vi "Interlock Chain Close Connections.vi"(8 "error in (no error)":errorcluster, 11 "CO2 Actor in":refnum<class "CO2 Actor.lvclass">) -> (0 "error out":errorcluster, 3 "CO2 Actor out":refnum<class "CO2 Actor.lvclass">)   [LabVIEW 2015, in "cRIO-Carbondioxide.lvlib" / "CO2-Actor.lvlib" / "CO2 Actor.lvclass"]
uses:
  CO2 Actor.lvclass
  CO2 Actor.lvclass/CO2 Actor.ctl
  Interlocks/Interlock Chain/Interlock Chain.lvclass/Interlock Chain.ctl
  Interlocks/Interlock/Interlock.lvclass
  Interlocks/Interlock Chain/Interlock Chain.lvclass
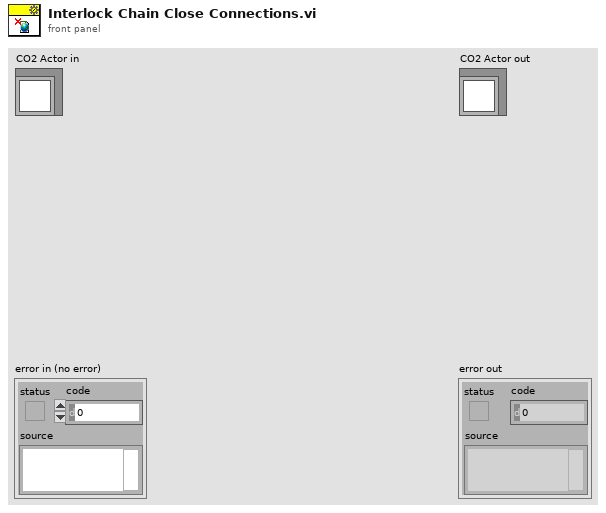
[diagram p1: front panel]
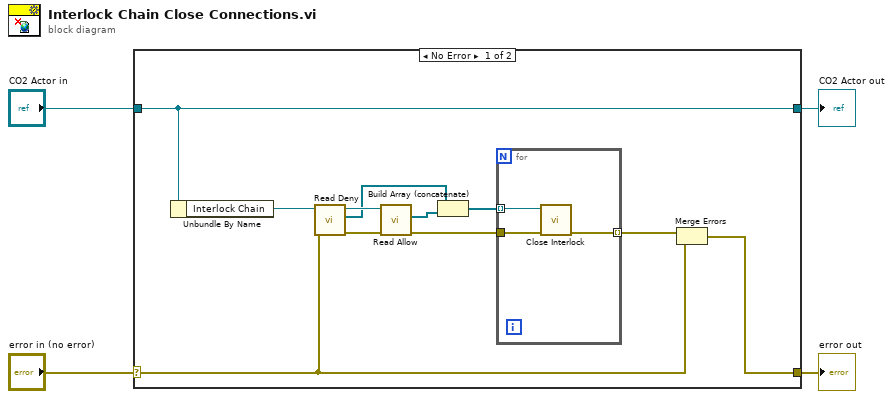
[diagram p0: block diagram]
diagram:
  n1 = case shown="No Error" "error in (no error)" {
    selector: "error in (no error)" -> [w11 w20]
    tunnel: [w13 w20] -> w3
    tunnel: [w15 w19] -> w1
    tunnel: "CO2 Actor in" -> [w15 w19]
    frame No Error {
      n2 = Unbundle By Name(w15) -> ("Interlock Chain"=w12:refnum<class "Interlock Chain.lvclass">)
      n3 = call "Read Deny.vi"("error in (no error)"=w11, "Interlock Chain in"=w12) -> ("error out"=w10:errorcluster, "Deny"=w5:refnum<class "Interlock.lvclass">[], "Interlock Chain out"=w9:refnum<class "Interlock Chain.lvclass">)  [unwired: 7 in]
      n4 = call "Read Allow.vi"("error in (no error)"=w10, "Interlock Chain in"=w9) -> ("error out"=w6:errorcluster, "Allow"=w8:refnum<class "Interlock.lvclass">[])  [unwired: 6 in, 2 out]
      n5 = Build Array (concatenate)(w5, w8) -> (w7:refnum<class "Interlock.lvclass">[])
      n6 = for {
        tunnel: w7 -> [w18] mode=indexing
        tunnel: w6 -> [w17]
        tunnel: [w16] -> w14 mode=indexing
        n7 = call-dynamic "Close Interlock.vi"("error in (no error)"=w17, "Interlock in"=w18) -> ("error out"=w16:errorcluster)  [unwired: 8 in, 1 out]
      }
      n8 = Merge Errors(w14, w11) -> (w13:errorcluster)
    }
    frame Error {
    }
  }
  "error out" <- w3
  "CO2 Actor out" <- w1
